vi "SaveDataFile.vi"(0 "Data Array":dbl[][](array[numeric]), 1 "Temperature":dbl, 2 "Run uninterrupted?":bool, 3 "Humidity":dbl, 5 "no. of arrays":i32, 9 "Actual array lengths":i32, 11 "Error In":errorcluster, 12 "Array Titles":string, 13 "Strip Segment":string, 14 "Arrays format":string) -> (4 "Filename OUT":string, 6 "Pathname OUT":string, 10 "Path + Filename OUT":string, 15 "Error Out":errorcluster)   [LabVIEW 2018]
uses:
  globals/QC_RunInformation.vi
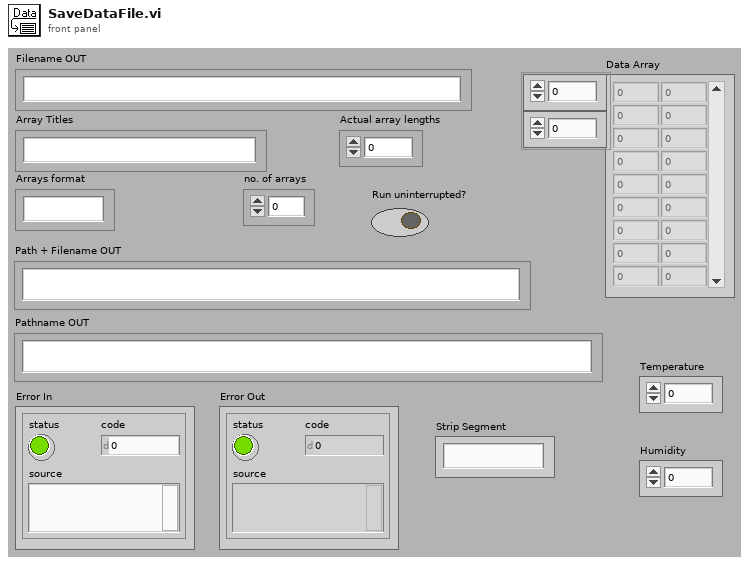
[diagram p1: front panel]
types:
  T1 = enum16{"open", "open or create", "create or replace", "create"}
  T2 = cluster{"Sensor Serial No.:":string, "Wafer:":string, "Batch:":string, "Manufacturer:":string, "Device Category:":string, "Database Serial No.:":string, "Date Initiated:":string, "Time Initiated:":string, "Test":string, "Probeplan used:":string, "End of Run comment:":string, "User:":string, "Vbias SMU":string, "LCR":string, "Test SMU":string, "Test DMM":string, "Comments":string}
  T3 = cluster{"Institute":string, "Manufacturers":string[], "Devices":string[], "Serialnumbers Lookup DB":string, "Data directory":string, "Backup & screenshot directory":string, "List of known users":string[], "Measurement switch not used":bool, "Measurement Switch":string, "DUT Switch":string, "Rseries IV [MOhm]":string, "Rshunt IV [MOhm]":string, "Rseries CV [MOhm]":string, "DC blocking Cap [µF]":string, "Rseries LCR [MOhm]":string, "Rseries stability [MOhm]":string, "Rshunt stability [MOhm]":string, "Rseries striptest bias [MOhm]":string, "Rseries strip pinhole [MOhm]":string}
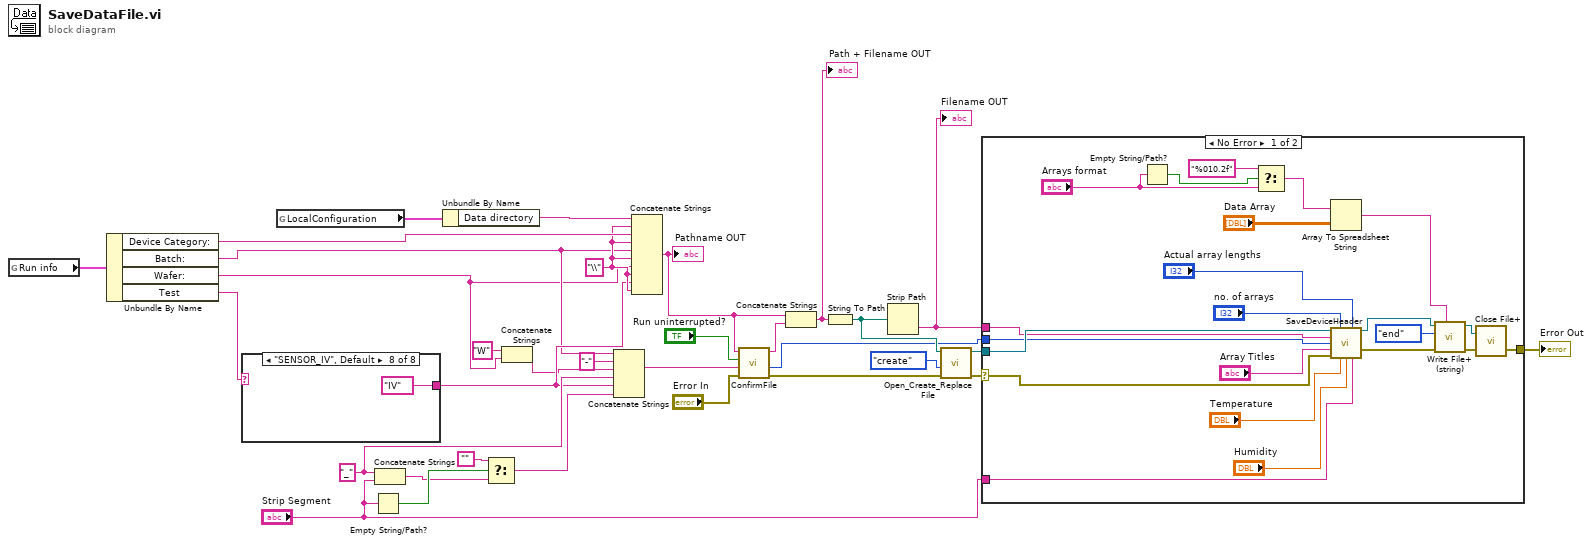
[diagram p0: block diagram]
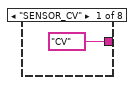
[diagram p2: hidden frame]
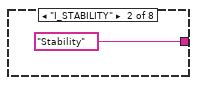
[diagram p3: hidden frame]
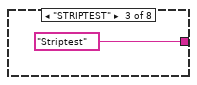
[diagram p4: hidden frame]
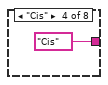
[diagram p5: hidden frame]
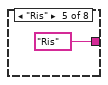
[diagram p6: hidden frame]
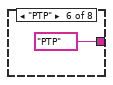
[diagram p7: hidden frame]
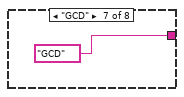
[diagram p8: hidden frame]
diagram:
  w13 = "_"
  w23 = "\\"
  n1 = global read "QC_RunInformation.vi" "Run info"() -> (w31:T2)
  n2 = Unbundle By Name(w31) -> ("Device Category:"=w29:string, "Batch:"=w5:string, "Wafer:"=w2:string, "Test"=w8:string)
  n3 = case shown="\"SENSOR_IV\", Default" w8 {
    tunnel: ["CV" ("Test") "Stability" ("Test") "Striptest" ("Test") "Cis" ("Test") "Ris" ("Test") "PTP" ("Test") "GCD" ("Test") "IV" ("Test")] -> w7
    frame "SENSOR_CV" {
    }
    frame "I_STABILITY" {
    }
    frame "STRIPTEST" {
    }
    frame "Cis" {
    }
    frame "Ris" {
    }
    frame "PTP" {
    }
    frame "GCD" {
    }
    frame "SENSOR_IV", Default {
    }
  }
  n4 = global read "QC_RunInformation.vi" "LocalConfiguration"() -> (w32:T3)
  n5 = Empty String/Path?(string/path="Strip Segment") -> (empty?=w15:bool)
  n6 = Concatenate Strings(w13, "Strip Segment") -> (w11:string)
  n7 = Unbundle By Name(w32) -> ("Data directory"=w30:string)
  n8 = Select(t="", s=w15, f=w11) -> (s? t:f=w12:string)
  n9 = Concatenate Strings("W" ("string"), w2) -> (w1:string)
  n10 = Concatenate Strings(w5, "-" ("string"), w1, w13, w7, w12) -> (w22:string)
  n11 = Concatenate Strings(w30, w23, w29, w23, w5, w23, w2, w23, w7, w23) -> (w18:string)
  "Pathname OUT" <- w18
  n12 = call "ConfirmFile.vi"("Error In"="Error In", "Filename IN"=w22, "Run uninterrupted?"="Run uninterrupted?", "Pathname IN"=w18) -> ("Error Out"=w19:errorcluster, "Run Number"=w10:i32, "Filename:"=w17:string)  [unwired: 1 in]
  n13 = Concatenate Strings(w18, w17) -> (w16:string)
  "Path + Filename OUT" <- w16
  n14 = String To Path(string=w16) -> (path=w25:path)
  n15 = Strip Path(path=w25) -> (name=w26:string)  [unwired: 1 out]
  "Filename OUT" <- w26
  n16 = call <vilib>:"Open_Create_Replace File.vi"("error in (no error)"=w19, "function (open:0)"=T1."create", "file path"=w25) -> ("error out"=w24:errorcluster, "refnum"=w27:refnum<file>)  [unwired: 5 in, 2 out]
  n17 = case shown="No Error" w24 {
    selector: w24 -> [w62 w63]
    tunnel: w27 -> [w51 _]
    tunnel: w26 -> [w50 _]
    tunnel: [w46 w63] -> w21
    tunnel: w10 -> [w42 _]
    tunnel: "Strip Segment" -> [w41 _]
    frame No Error {
      n18 = Empty String/Path?(string/path="Arrays format") -> (empty?=w59:bool)
      n19 = Select(t="%010.2f", s=w59, f="Arrays format") -> (s? t:f=w57:string)
      n20 = Array To Spreadsheet String(array="Data Array", 3:w57) -> (spreadsheet string=w56:string)  [unwired: 1 in]
      n21 = call "SaveDeviceHeader.vi"("File Refnum in"=w51, "no. of arrays"="no. of arrays", "Array Lengths"="Actual array lengths", "Filename"=w50, "Run Number"=w42, "Array Titles"="Array Titles", "error in (no error)"=w62, "Temperature"="Temperature", "Humidity"="Humidity", "Strip Segment"=w41) -> ("File Refnum out"=w52:refnum<file>, "error out"=w43:errorcluster)  [unwired: 3 in, 1 out]
      n22 = call <vilib>:"Write File+ (string).vi"("string"=w56, "error in (no error)"=w43, "pos mode (rel. to end:1)"=enum16{"start", "end", "current"}."end", "refnum"=w52) -> ("error out"=w55:errorcluster, "dup refnum"=w53:refnum<file>)  [unwired: 3 in, 1 out]
      n23 = call <vilib>:"Close File+.vi"("error in (no error)"=w55, "refnum"=w53) -> ("error out"=w46:errorcluster)  [unwired: 3 in, 2 out]
    }
    frame Error {
    }
  }
  "Error Out" <- w21
